vi "Results to String.vi"(11 "Results":T1) -> (3 "Results String":string)   [LabVIEW 2020]
uses:
  IA dbg/Inflation-Apparatus/src/Controls/Outputs.ctl
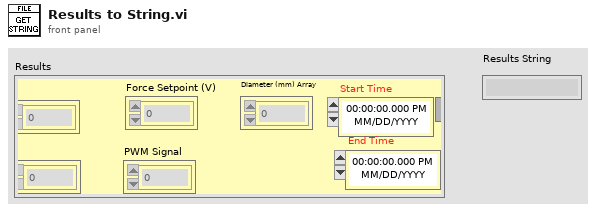
[diagram p1: front panel]
types:
  T1 = typedef "Outputs.ctl" = cluster{"Force Setpoint (V)":dbl[], "PWM Signal":dbl[], "Diameter (mm) Array":dbl[], "Force (V)":dbl[], "Force Time (s)":dbl[], "Start Time":timestamp, "End Time":timestamp}
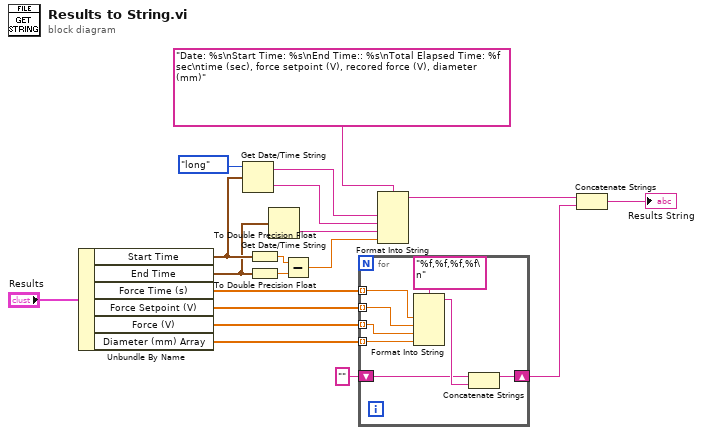
[diagram p0: block diagram]
diagram:
  n1 = Unbundle By Name("Results") -> ("Start Time"=w14:timestamp, "End Time"=w9:timestamp, "Force Time (s)"=w8:dbl[], "Force Setpoint (V)"=w7:dbl[], "Force (V)"=w6:dbl[], "Diameter (mm) Array"=w5:dbl[])
  n2 = Get Date/Time String(date format (0)=enum16{"short", "long", "abbreviated"}."long", seconds (now)=w14) -> (date string=w12:string, time string=w11:string)  [unwired: 1 in]
  n3 = To Double Precision Float(number=w14) -> (double precision float=w16:dbl)
  n4 = To Double Precision Float(number=w9) -> (double precision float=w17:dbl)
  n5 = Get Date/Time String(seconds (now)=w9) -> (time string=w10:string)  [unwired: 2 in, 1 out]
  n6 = Subtract(x=w16, y=w17) -> (x-y=w15:dbl)
  n7 = for {
    tunnel: w8 -> [w24] mode=indexing
    tunnel: w7 -> [w25] mode=indexing
    tunnel: w6 -> [w26] mode=indexing
    tunnel: w5 -> [w27] mode=indexing
    shift-right: [w21] -> w2
    shift-left: "" -> [w20]
    n8 = Format Into String(format string="%f,%f,%f,%f\n", w24, w25, w26, w27) -> (resulting string=w22:string)  [unwired: 2 in, 1 out]
    n9 = Concatenate Strings(w20, w22) -> (w21:string)
  }
  n10 = Format Into String(format string="Date: %s\nStart Time: %s\nEnd Time:: %s\nTotal Elapsed Time: %f sec\ntime (sec), force setpoint (V), recored force (V), diameter (mm)", w12, w11, w10, w15) -> (resulting string=w3:string)  [unwired: 2 in, 1 out]
  n11 = Concatenate Strings(w3, w2) -> (→"Results String":string)
